vi "Auth_Token.vi"(6 "Token header key (Authorization)":string, 7 "Token empty preamble (False)":bool, 8 "error in (no error)":errorcluster, 9 "Token preamble (Token)":string="Token", 10 "Token":string, 11 "ByteGSAPIBase in":refnum<class "RESTBase.lvclass">) -> (0 "error out":errorcluster, 3 "ByteGSAPIBase out":refnum<class "RESTBase.lvclass">)   [LabVIEW 2019, in "ByteREST.lvlib" / "RESTBase.lvclass"]
doc: "Apre una nuova connessione HTTP e setta il content type a \"application/json\""
uses:
  RESTBase.lvclass
  RESTBase.lvclass/RESTBase.ctl
  <vilib>/httpClient/LabVIEWHTTPClient.lvlib
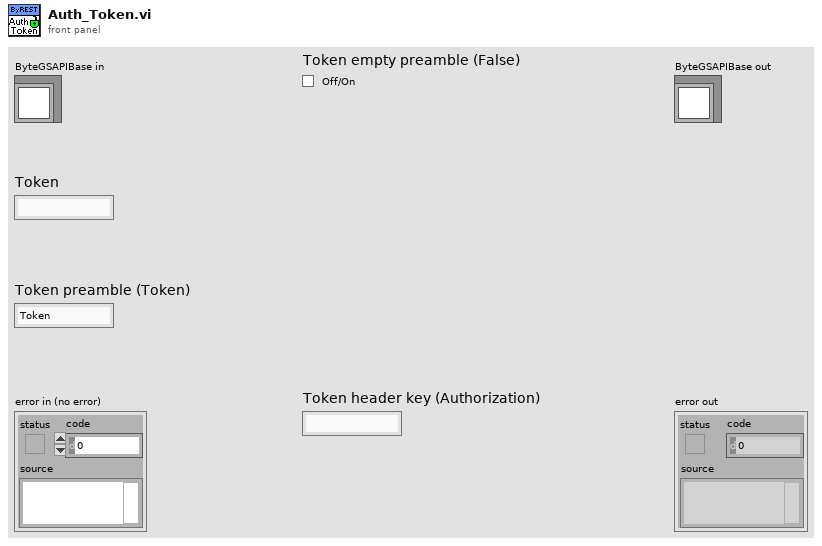
[diagram p1: front panel]
types:
  T1 = typedef "LabVIEWHTTPClient.lvlib/ClientHandle.ctl" = refnum<k1>
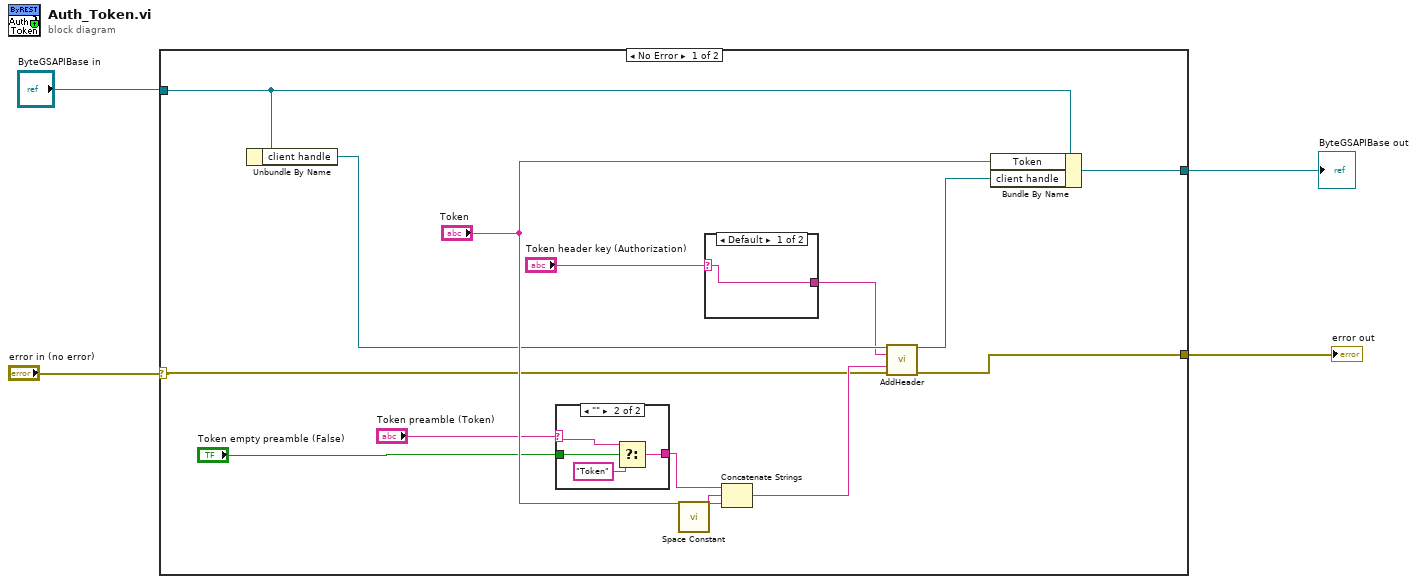
[diagram p0: block diagram]
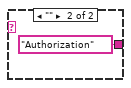
[diagram p3: hidden frame]
diagram:
  n1 = case shown="No Error" "error in (no error)" {
    selector: "error in (no error)" -> [w13 w27]
    tunnel: [w15 w27] -> w3
    tunnel: [w18 w26] -> w1
    tunnel: "ByteGSAPIBase in" -> [w12 w26]
    frame No Error {
      n2 = Unbundle By Name(w12) -> ("client handle"=w11:T1)
      n3 = case shown="\"\"" "Token preamble (Token)" {
        selector: "Token preamble (Token)" -> [w19 w21]
        tunnel: [w19 w23] -> w6
        tunnel: "Token empty preamble (False)" -> [_ w20]
        frame Default {
        }
        frame "" {
          n4 = Select(t=w21, s=w20, f="Token") -> (s? t:f=w23:string)
        }
      }
      n5 = call <vilib>:"Space Constant.vi"() -> ("String"=w10:string)
      n6 = case shown="Default" "Token header key (Authorization)" {
        selector: "Token header key (Authorization)" -> [w24 _]
        tunnel: [w24 "Authorization" ("header")] -> w8
        frame Default {
        }
        frame "" {
        }
      }
      n7 = Concatenate Strings(w6, w10, "Token") -> (w17:string)
      n8 = call <vilib>:"AddHeader.vi"("client handle"=w11, "header"=w8, "value"=w17, "error in (no error)"=w13) -> ("client handle out"=w14:T1, "error out"=w15:errorcluster)  [unwired: 10 in]
      n9 = Bundle By Name(cluster=w12, "Token"="Token", "client handle"=w14) -> (w18:refnum<class "RESTBase.lvclass">)
    }
    frame Error {
    }
  }
  "error out" <- w3
  "ByteGSAPIBase out" <- w1
